vi "Save Data D (SubVI).vi"(0 "Save Enable":bool, 5 "Save Interval [s]":dbl=1.0 min=0.0, 7 "File Name":string, 9 "Folder Location":path, 11 "Data Array (Row)":string[](array[string]), 12 "Column Header Array":string[](array[string]), 13 "Title Block":string[][](array[string]), 14 "External Save Signal":bool) -> (4 "File Path":path, 8 "Save Indicator LED":bool, 15 "Save Error":errorcluster)   [LabVIEW 2011]
panel:
  in  "Error Input":errorcluster
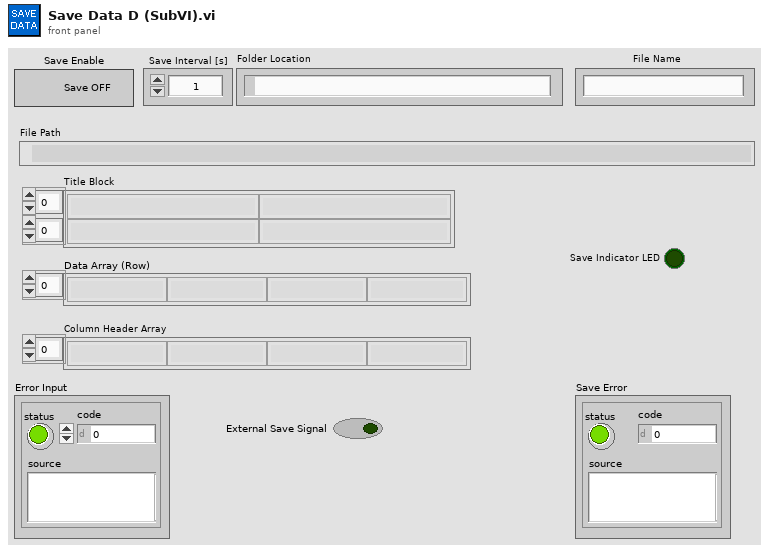
[diagram p1: front panel]
types:
  T1 = enum16{"open", "replace", "create", "open or create", "replace or create", "replace or create with confirmation"}
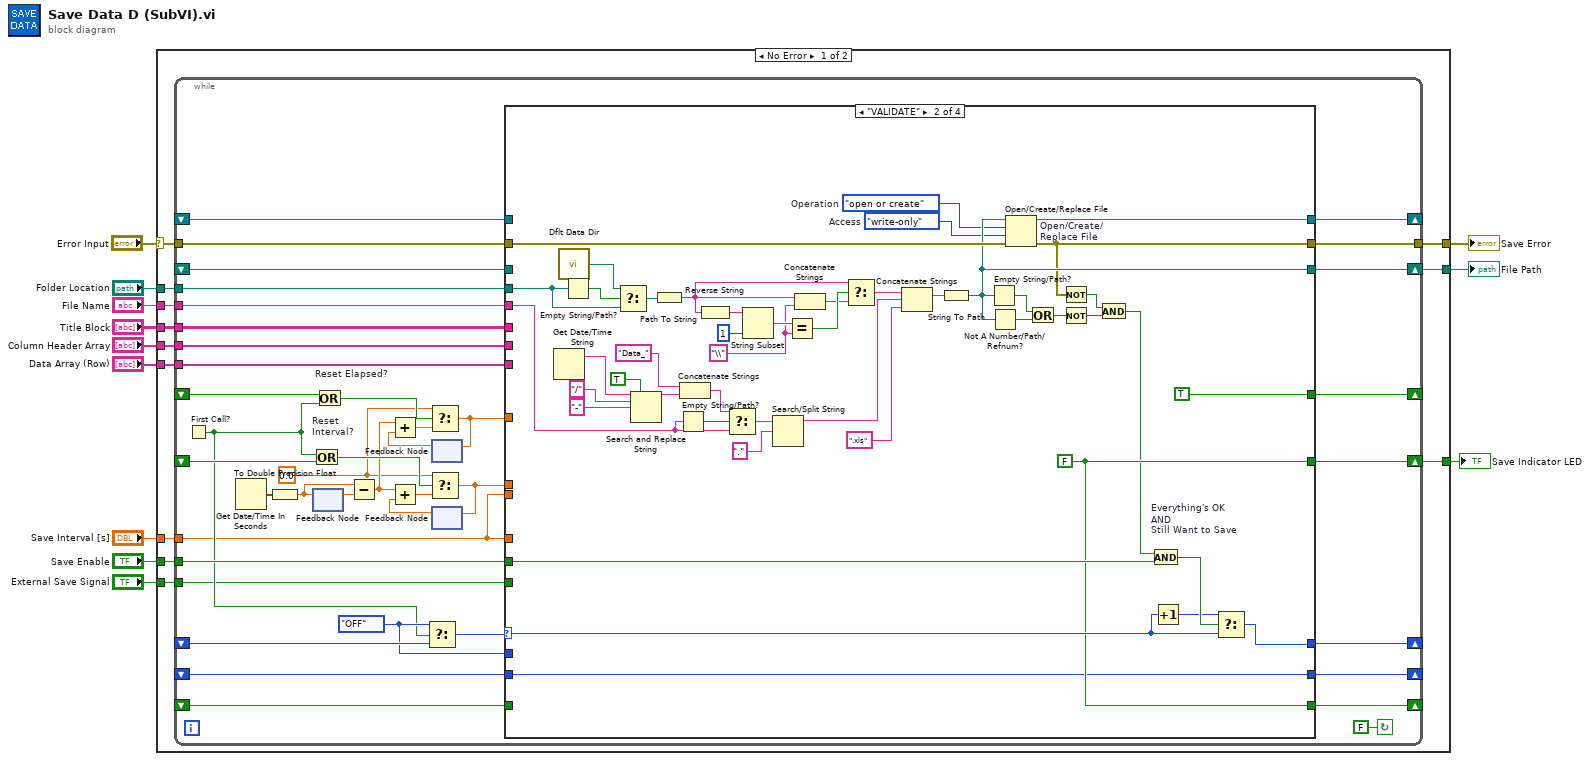
[diagram p0: block diagram]
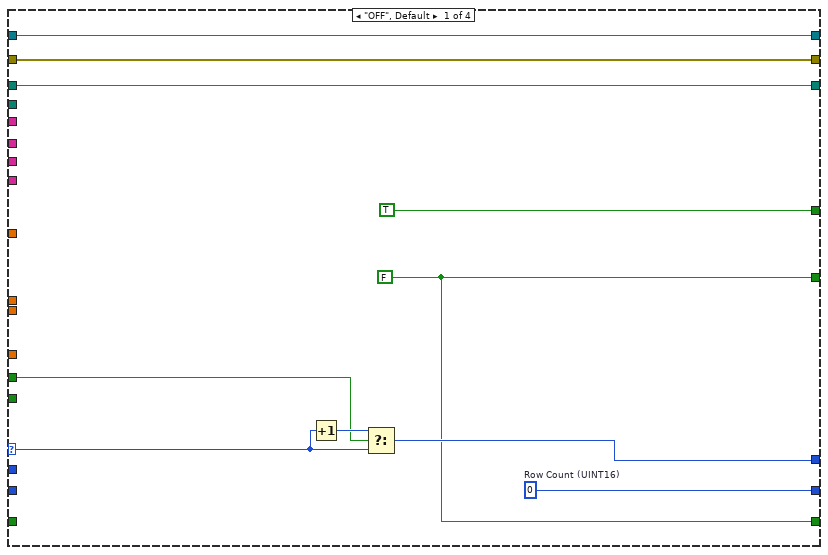
[diagram p2: hidden frame]
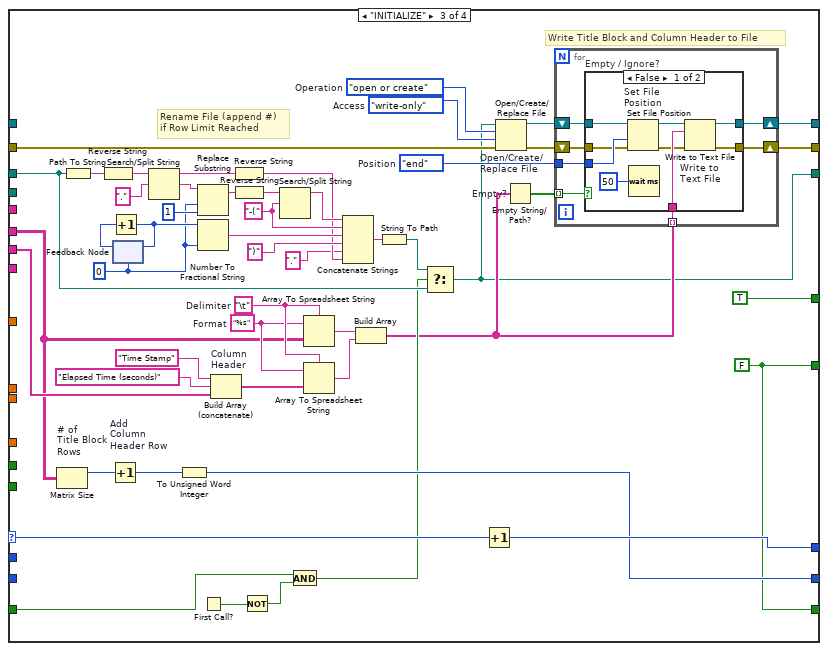
[diagram p3: hidden frame]
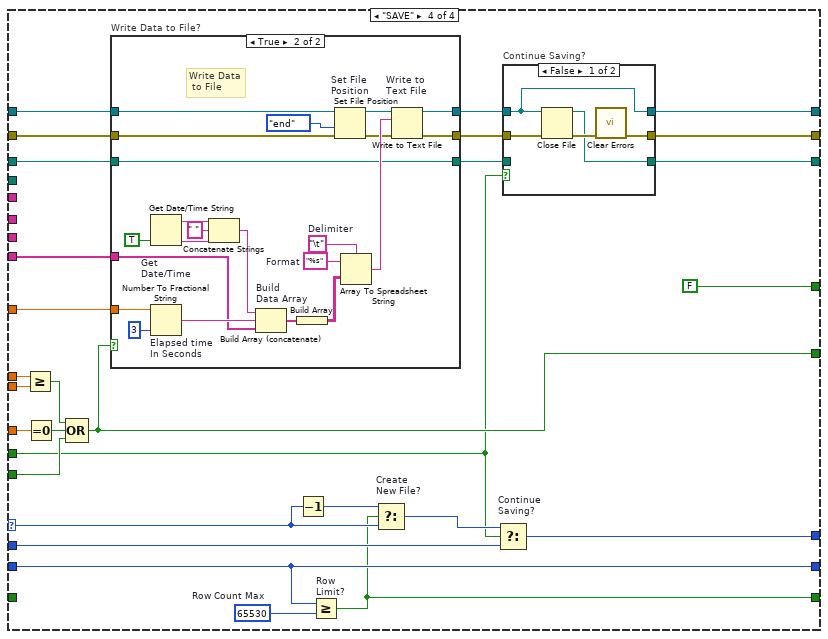
[diagram p5: hidden frame]
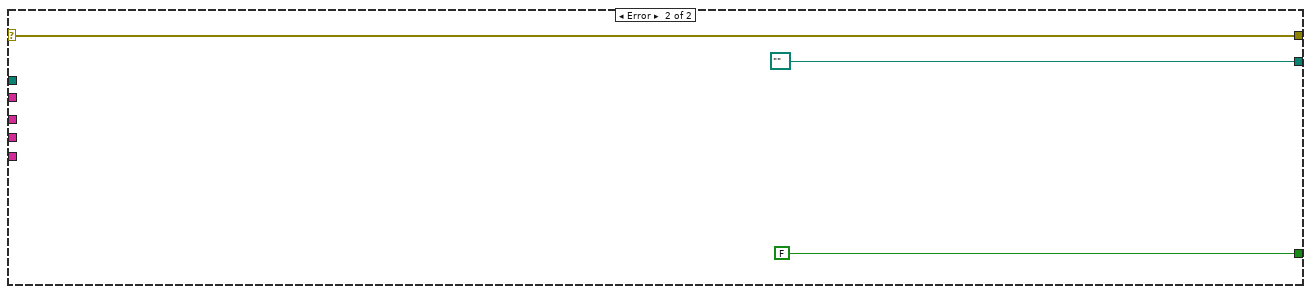
[diagram p8: hidden frame]
diagram:
  n1 = case shown="No Error" "Error Input" {
    selector: "Error Input" -> [w14 w253]
    tunnel: "Title Block" -> [w24 _]
    tunnel: "Column Header Array" -> [w23 _]
    tunnel: "Data Array (Row)" -> [w22 _]
    tunnel: "Save Interval [s]" -> [w21 _]
    tunnel: "Save Enable" -> [w20 _]
    tunnel: "Folder Location" -> [w19 _]
    tunnel: "File Name" -> [w18 _]
    tunnel: "External Save Signal" -> [w17 _]
    tunnel: [w16 w253] -> w11
    tunnel: [w15 path "" ("path")] -> w2
    tunnel: [w13 FALSE] -> w1
    frame No Error {
      n2 = while {
        tunnel: w20 -> [w33]
        shift-right: [w62] -> _
        shift-left: _ -> [w64]
        shift-right: [w60] -> _
        shift-left: _ -> [w59]
        tunnel: w24 -> [w58]
        tunnel: w23 -> [w57]
        tunnel: w14 -> [w56]
        tunnel: w22 -> [w55]
        shift-right: [w54] -> w15
        shift-left: _ -> [w53]
        shift-right: [w52] -> _
        shift-left: _ -> [w51]
        shift-right: [w38] -> _
        shift-left: _ -> [w35]
        shift-right: [w37] -> w13
        shift-left: _ -> [w36]
        tunnel: w21 -> [w29]
        tunnel: w19 -> [w32]
        tunnel: w18 -> [w30]
        tunnel: w17 -> [w28]
        tunnel: [w27] -> w16
        shift-right: [w26] -> _
        shift-left: _ -> [w25]
        stop <- FALSE continue-if-true
        w39 = 0.0 ("t")
        w61 = enum16{"OFF", "VALIDATE", "INITIALIZE", "SAVE"}."OFF"
        n3 = First Call?() -> (First Call?: T/F=w31:bool)
        n4 = Get Date/Time In Seconds() -> (seconds since 1Jan1904=w48:timestamp)
        n5 = To Double Precision Float(number=w48) -> (double precision float=w44:dbl)
        n6 = Or "Reset\nInterval?"(x=w31, y=w36) -> (x .or. y?=w46:bool)
        n7 = feedback #1() -> (w49:dbl)  [unwired: 1 in]
        n8 = feedback-in #1(w44) -> ()
        n9 = Or "Reset Elapsed?"(x=w35, y=w31) -> (x .or. y?=w43:bool)
        n10 = Subtract(x=w44, y=w49) -> (x-y=w40:dbl)
        n11 = Select(t=w61, s=w31, f=w64) -> (s? t:f=w63:enum16{"OFF", "VALIDATE", "INITIALIZE", "SAVE"})
        n12 = feedback #2() -> (w41:dbl)  [unwired: 1 in]
        n13 = Add(x=w40, y=w41) -> (x+y=w45:dbl)
        n14 = Select(t=w39, s=w43, f=w45) -> (s? t:f=w50:dbl)
        n15 = feedback-in #2(w50) -> ()
        n16 = feedback #3() -> (w42:dbl)  [unwired: 1 in]
        n17 = Add(x=w40, y=w42) -> (x+y=w47:dbl)
        n18 = Select(t=w39, s=w46, f=w47) -> (s? t:f=w34:dbl)
        n19 = feedback-in #3(w34) -> ()
        n20 = case shown="\"VALIDATE\"" w63 {
          selector: w63 -> [w73 w118 w172 w210]
          tunnel: [w71 w117 w171 w218] -> w62
          tunnel: w33 -> [w72 w121 _ w197]
          tunnel: w61 -> [_ _ _ w217]
          tunnel: [w67 w102 w158 w212] -> w60
          tunnel: w59 -> [_ w102 _ w212]
          tunnel: w58 -> [_ _ w161 _]
          tunnel: w53 -> [w75 _ w157 w198]
          tunnel: w57 -> [_ _ w166 _]
          tunnel: w56 -> [w70 w109 w127 w214]
          tunnel: w55 -> [_ _ _ w215]
          tunnel: w50 -> [_ _ _ w216]
          tunnel: [w75 w108 w122 w192] -> w54
          tunnel: [w68 w115 w132 w208] -> w52
          tunnel: w51 -> [_ _ w153 _]
          tunnel: [TRUE TRUE TRUE FALSE] -> w38
          tunnel: [w68 w115 w132 w200] -> w37
          tunnel: w34 -> [_ _ _ w206]
          tunnel: w29 -> [_ _ _ w205]
          tunnel: w32 -> [_ w77 _ _]
          tunnel: w30 -> [_ w80 _ _]
          tunnel: w29 -> [_ _ _ w204]
          tunnel: w28 -> [_ _ _ w201]
          tunnel: [w70 w107 w131 w194] -> w27
          tunnel: [w66 w100 w125 w191] -> w26
          tunnel: w25 -> [w66 _ _ w199]
          frame "OFF", Default {
            w67 = u16 0  # Row Count (UINT16)
            w68 = FALSE
            n21 = Increment(x=w73) -> (x+1=w74:enum16{"OFF", "VALIDATE", "INITIALIZE", "SAVE"})
            n22 = Select(t=w74, s=w72, f=w73) -> (s? t:f=w71:enum16{"OFF", "VALIDATE", "INITIALIZE", "SAVE"})
          }
          frame "VALIDATE" {
            w99 = enum16{"read/write", "read-only", "write-only"}."write-only"  # Access
            w98 = T1."open or create"  # Operation
            w84 = "\\"
            w115 = FALSE
            n23 = Get Date/Time String() -> (date string=w94:string)  [unwired: 3 in, 1 out]
            n24 = call <vilib>:"Dflt Data Dir.vi"() -> ("App:Default Data Directory"=w78:path)
            n25 = Empty String/Path?(string/path=w77) -> (empty?=w81:bool)
            n26 = Select(t=w78, s=w81, f=w77) -> (s? t:f=w79:path)
            n27 = Search and Replace String(replace all?=TRUE, input string=w94, search string="/", replace string="-") -> (result string=w91:string)  [unwired: 4 in, 3 out]
            n28 = Path To String(path=w79) -> (string=w76:string)
            n29 = Empty String/Path?(string/path=w80) -> (empty?=w97:bool)
            n30 = Concatenate Strings("Data_" ("search string/char (-)"), w91) -> (w90:string)
            n31 = Reverse String(1:w76) -> (0:w88:string)
            n32 = Select(t=w90, s=w97, f=w80) -> (s? t:f=w89:string)
            n33 = String Subset(string=w88, length (rest)=1) -> (substring=w86:string)  [unwired: 1 in]
            n34 = Search/Split String(string=w89, search string/char (-)=".") -> (substring before match=w103:string)  [unwired: 1 in, 2 out]
            n35 = Equal?(x=w86, y=w84) -> (x = y?=w85:bool)
            n36 = Concatenate Strings(w76, w84) -> (w83:string)
            n37 = Select(t=w76, s=w85, f=w83) -> (s? t:f=w82:string)
            n38 = Concatenate Strings(w82, w103, ".xls" ("string")) -> (w113:string)
            n39 = String To Path(string=w113) -> (path=w108:path)
            n40 = Empty String/Path?(string/path=w108) -> (empty?=w112:bool)
            n41 = Not A Number/Path/Refnum?(number/path/refnum=w108) -> (NaN/Path/Refnum?=w111:bool)
            n42 = Open/Create/Replace File "Open/Create/\nReplace File"(file path (use dialog)=w108, error in=w109, operation (0:open)=w98, access (0:read/write)=w99) -> (refnum out=w100:refnum<file>, error out=w107:errorcluster)  [unwired: 2 in, 1 out]
            n43 = Or(x=w112, y=w111) -> (x .or. y?=w110:bool)
            n44 = Not(x=w107) -> (.not. x?=w106:bool)
            n45 = Not(x=w110) -> (.not. x?=w105:bool)
            n46 = And(x=w106, y=w105) -> (x .and. y?=w101:bool)
            n47 = And "Everything's OK\nAND\nStill Want to Save"(x=w101, y=w121) -> (x .and. y?=w120:bool)
            n48 = Increment(x=w118) -> (x+1=w119:enum16{"OFF", "VALIDATE", "INITIALIZE", "SAVE"})
            n49 = Select(t=w119, s=w120, f=w118) -> (s? t:f=w117:enum16{"OFF", "VALIDATE", "INITIALIZE", "SAVE"})
          }
          frame "INITIALIZE" {
            w129 = enum16{"read/write", "read-only", "write-only"}."write-only"  # Access
            w134 = u8 0
            w142 = "-("
            w132 = FALSE
            w162 = enum16{"start", "end", "current"}."end"  # Position
            w130 = T1."open or create"  # Operation
            w170 = "\t"  # Delimiter
            w169 = "%s"  # Format
            # "Rename File (append #)\nif Row Limit Reached"
            # "Write Title Block and Column Header to File"
            n50 = Matrix Size "# of\nTitle Block\nRows"(0:w161) -> (1:w160:i32)  [unwired: 1 out]
            n51 = Path To String(path=w157) -> (string=w145:string)
            n52 = Reverse String(1:w145) -> (0:w146:string)
            n53 = Increment "Add\nColumn\nHeader Row"(x=w160) -> (x+1=w159:i32)
            n54 = feedback #4(w134) -> (w140:u8)
            n55 = Increment(x=w140) -> (x+1=w141:u8)
            n56 = feedback-in #4(w141) -> ()
            n57 = Search/Split String(string=w146, search string/char (-)=".") -> (substring before match=w147:string, match + rest of string=w148:string)  [unwired: 2 out]
            n58 = To Unsigned Word Integer(number=w159) -> (unsigned 16bit integer=w158:u16)
            n59 = Replace Substring(2:1 ("length (len. of substring)"), 3:w134, 5:w148) -> (1:w149:string)  [unwired: 2 out]
            n60 = Number To Fractional String(number=w141, precision (6)=w134) -> (F-format string=w151:string)  [unwired: 2 in]
            n61 = First Call?() -> (First Call?: T/F=w152:bool)
            n62 = Build Array (concatenate) "Column\nHeader"("Time Stamp", "Elapsed Time (seconds)", w166) -> (w165:string[])
            n63 = Reverse String(1:w147) -> (0:w137:string)
            n64 = Reverse String(1:w149) -> (0:w143:string)
            n65 = Not(x=w152) -> (.not. x?=w155:bool)
            n66 = Search/Split String(string=w143, search string/char (-)=w142) -> (substring before match=w139:string)  [unwired: 1 in, 2 out]
            n67 = And(x=w153, y=w155) -> (x .and. y?=w154:bool)
            n68 = Array To Spreadsheet String(delimiter (Tab)=w170, array=w161, 3:w169) -> (spreadsheet string=w164:string)
            n69 = Array To Spreadsheet String(delimiter (Tab)=w170, array=w165, 3:w169) -> (spreadsheet string=w163:string)
            n70 = Concatenate Strings(w139, w142, w151, ")", "." ("search string/char (-)"), w137) -> (w136:string)
            n71 = Build Array(w164, w163) -> (w124:string[])
            n72 = String To Path(string=w136) -> (path=w156:path)
            n73 = Select ("Rename File\nIF Row Limit\nReached")(t=w156, s=w154, f=w157) -> (s? t:f=w122:path)
            n74 = Increment(x=w172) -> (x+1=w171:enum16{"OFF", "VALIDATE", "INITIALIZE", "SAVE"})
            n75 = Open/Create/Replace File "Open/Create/\nReplace File"(file path (use dialog)=w122, error in=w127, operation (0:open)=w130, access (0:read/write)=w129) -> (refnum out=w128:refnum<file>, error out=w126:errorcluster)  [unwired: 2 in, 1 out]
            n76 = Empty String/Path? "Empty?"(string/path=w124) -> (empty?=w123:bool[])
            n77 = for {
              tunnel: w124 -> [w178] mode=indexing
              tunnel: w162 -> [w177]
              shift-right: [w179] -> w131
              shift-left: w126 -> [w176]
              shift-right: [w174] -> w125
              shift-left: w128 -> [w175]
              tunnel: w123 -> [w173] mode=indexing
              n78 = case "Empty / Ignore?" shown="False" w173 {
                tunnel: [w187 w190] -> w179
                tunnel: [w186 w189] -> w174
                tunnel: w178 -> [w185 _]
                tunnel: w177 -> [w184 _]
                tunnel: w176 -> [w183 w190]
                tunnel: w175 -> [w182 w189]
                frame False {
                  n79 = Set File Position "Set File \nPosition"(refnum=w182, from (0:start)=w184, error in=w183) -> (refnum out=w180:refnum<file>, error out=w181:errorcluster)  [unwired: 1 in]
                  n80 = Wait (ms)(milliseconds to wait=u32 50) -> ()  [unwired: 1 out]
                  n81 = Write to Text File "Write to \nText File"(file (use dialog)=w180, text=w185, error in=w181) -> (refnum out=w186:refnum<file>, error out=w187:errorcluster)  [unwired: 1 in, 1 out]
                }
                frame True {
                }
              }
            }
          }
          frame "SAVE" {
            w213 = u16 65530  # Row Count Max
            n82 = Greater Or Equal?(x=w206, y=w205) -> (x >= y?=w203:bool)
            n83 = Equal To 0?(x=w204) -> (x = 0?=w202:bool)
            n84 = Compound Arithmetic op=OR(w203, w202, w201) -> (w200:bool)
            n85 = case "Write Data to File?" shown="True" w200 {
              tunnel: w216 -> [_ w241]
              tunnel: w215 -> [_ w239]
              tunnel: w214 -> [w229 w236]
              tunnel: [w229 w235] -> w195
              tunnel: w199 -> [w227 w234]
              tunnel: w198 -> [w228 w231]
              tunnel: [w228 w231] -> w193
              tunnel: [w227 w230] -> w196
              frame False {
              }
              frame True {
                w238 = "\t"  # Delimiter
                w243 = "%s"  # Format
                # "Write Data\n to File"
                n86 = Get Date/Time String "Get \nDate/Time"(want seconds? (F)=TRUE) -> (date string=w244:string, time string=w247:string)  [unwired: 2 out]
                n87 = Number To Fractional String "Elapsed time\nIn Seconds"(number=w241, precision (6)=i16 3) -> (F-format string=w240:string)  [unwired: 2 in]
                n88 = Concatenate Strings(w244, " " ("string"), w247) -> (w248:string)
                n89 = Build Array (concatenate) "Build\nData Array"(w248, w240, w239) -> (w249:string[])
                n90 = Build Array(w249) -> (w250:string[][])
                n91 = Set File Position "Set File \nPosition"(refnum=w234, from (0:start)=enum16{"start", "end", "current"}."end", error in=w236) -> (refnum out=w232:refnum<file>, error out=w233:errorcluster)  [unwired: 1 in]
                n92 = Array To Spreadsheet String(delimiter (Tab)=w238, array=w250, 3:w243) -> (spreadsheet string=w237:string)
                n93 = Write to Text File "Write to \nText File"(file (use dialog)=w232, text=w237, error in=w233) -> (refnum out=w230:refnum<file>, error out=w235:errorcluster)  [unwired: 1 in, 1 out]
              }
            }
            n94 = Decrement(x=w210) -> (x-1=w211:enum16{"OFF", "VALIDATE", "INITIALIZE", "SAVE"})
            n95 = Greater Or Equal? "Row\nLimit?"(x=w212, y=w213) -> (x >= y?=w208:bool)
            n96 = Select "Create\nNew File?"(t=w211, s=w208, f=w210) -> (s? t:f=w209:enum16{"OFF", "VALIDATE", "INITIALIZE", "SAVE"})
            n97 = Select "Continue\nSaving?"(t=w209, s=w197, f=w217) -> (s? t:f=w218:enum16{"OFF", "VALIDATE", "INITIALIZE", "SAVE"})
            n98 = case "Continue Saving?" shown="False" w197 {
              tunnel: w196 -> [w219 w224]
              tunnel: w195 -> [w223 w225]
              tunnel: [w221 w225] -> w194
              tunnel: w193 -> [_ w226]
              tunnel: [w220 w226] -> w192
              tunnel: [w219 w224] -> w191
              frame False {
                n99 = Close File(refnum=w219, error in=w223) -> (path=w220:path, error out=w222:errorcluster)
                n100 = call <vilib>:"Clear Errors.vi"("error in (no error)"=w222) -> ("error out"=w221:errorcluster)  [unwired: 6 in]
              }
              frame True {
              }
            }
          }
        }
      }
    }
    frame Error {
    }
  }
  "Save Error" <- w11
  "File Path" <- w2
  "Save Indicator LED" <- w1
